vi "Answer.vi"(4 "连接ID":refnum<k5>, 6 "VISA串口名称":refnum<visa-resource-name>, 8 "error in (no error)":errorcluster caption="错误输入（无错误）", 9 "识别键":string, 10 "接收报文":string, 11 "MainPage 输入":refnum<class "MainPage.lvclass">) -> (0 "error out":errorcluster caption="错误输出", 3 "MainPage 输出":refnum<class "MainPage.lvclass">)   [LabVIEW 2019, in "MainPage.lvlib" / "MainPage.lvclass"]
uses:
  MainPage.lvclass
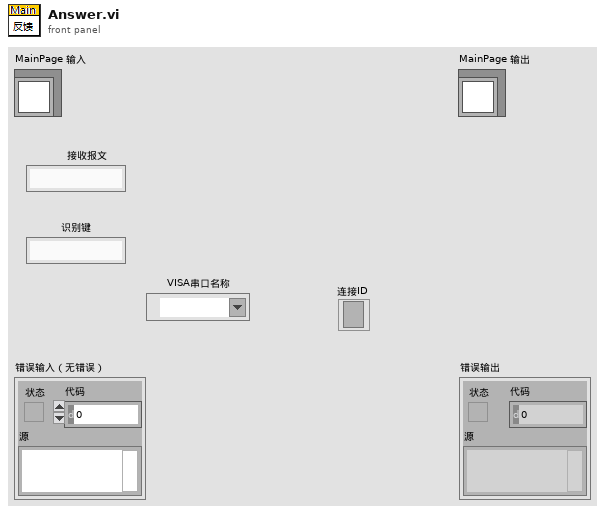
[diagram p1: front panel]
types:
  T1 = cluster{"类别":string, "通讯地址 U8":u8, "功能码 U8":u8, "寄存器地址 U16":u16, "数据/值 U16":u16, "16数据 U16":u16[]}
  T2 = cluster{"串口正常？":bool, "寄存器模拟":u16[], "报文信息记录":string[][]}
  T3 = enum16{"ini", "读取", "写入-报文记录", "写入-寄存器模拟", "写入-串口状态", "增加报文记录"}
  T4 = cluster{"寄存器模拟":u16[], "串口正常？":bool, "报文信息记录":string[][]}
  T5 = enum16{"ini", "增加记录", "读取记录", "更改寄存器值", "更改接口状态", "更改报文信息", "增加报文信息"}
  T6 = typedef "MainPage.lvlib/MainPage.lvclass/DataRef_通讯接口.ctl" = cluster{"连接方式":enum16{"网口(客服端)", "网口(服务端)", "串口"}, "VISA串口名称":refnum<visa-resource-name>, "服务端识别":cluster{"本机IP":string, "本机端口":u16, "当前目标":string}, "客服端识别":cluster{"客P-主IP:Port":string}, "服务端记录":cluster{"服务端侦听ID":refnum<k5>, "服务端接口记录":map{string, refnum<k5>}}, "客服端记录":map{string, refnum<k5>}}
  T7 = typedef "MainPage.lvlib/MainPage.lvclass/通用配置选项.ctl" = cluster{"ModBusRTU反馈":enum32{"模拟反馈", "无反馈", "错误反馈"}, "侦听周期":u32, "跳转反馈":bool, "报文记录数量":u16, "客服端新增模式":enum32{"单端模式", "多端共存"}}
  T8 = cluster{"类别":string, "通讯地址 U8":u8, "功能码 U8":u8, "03字节数 U8":u8, "03数据 U8":u8[], "6/16寄存器地址 U16":u16, "6/16数量/值 U16":u16}
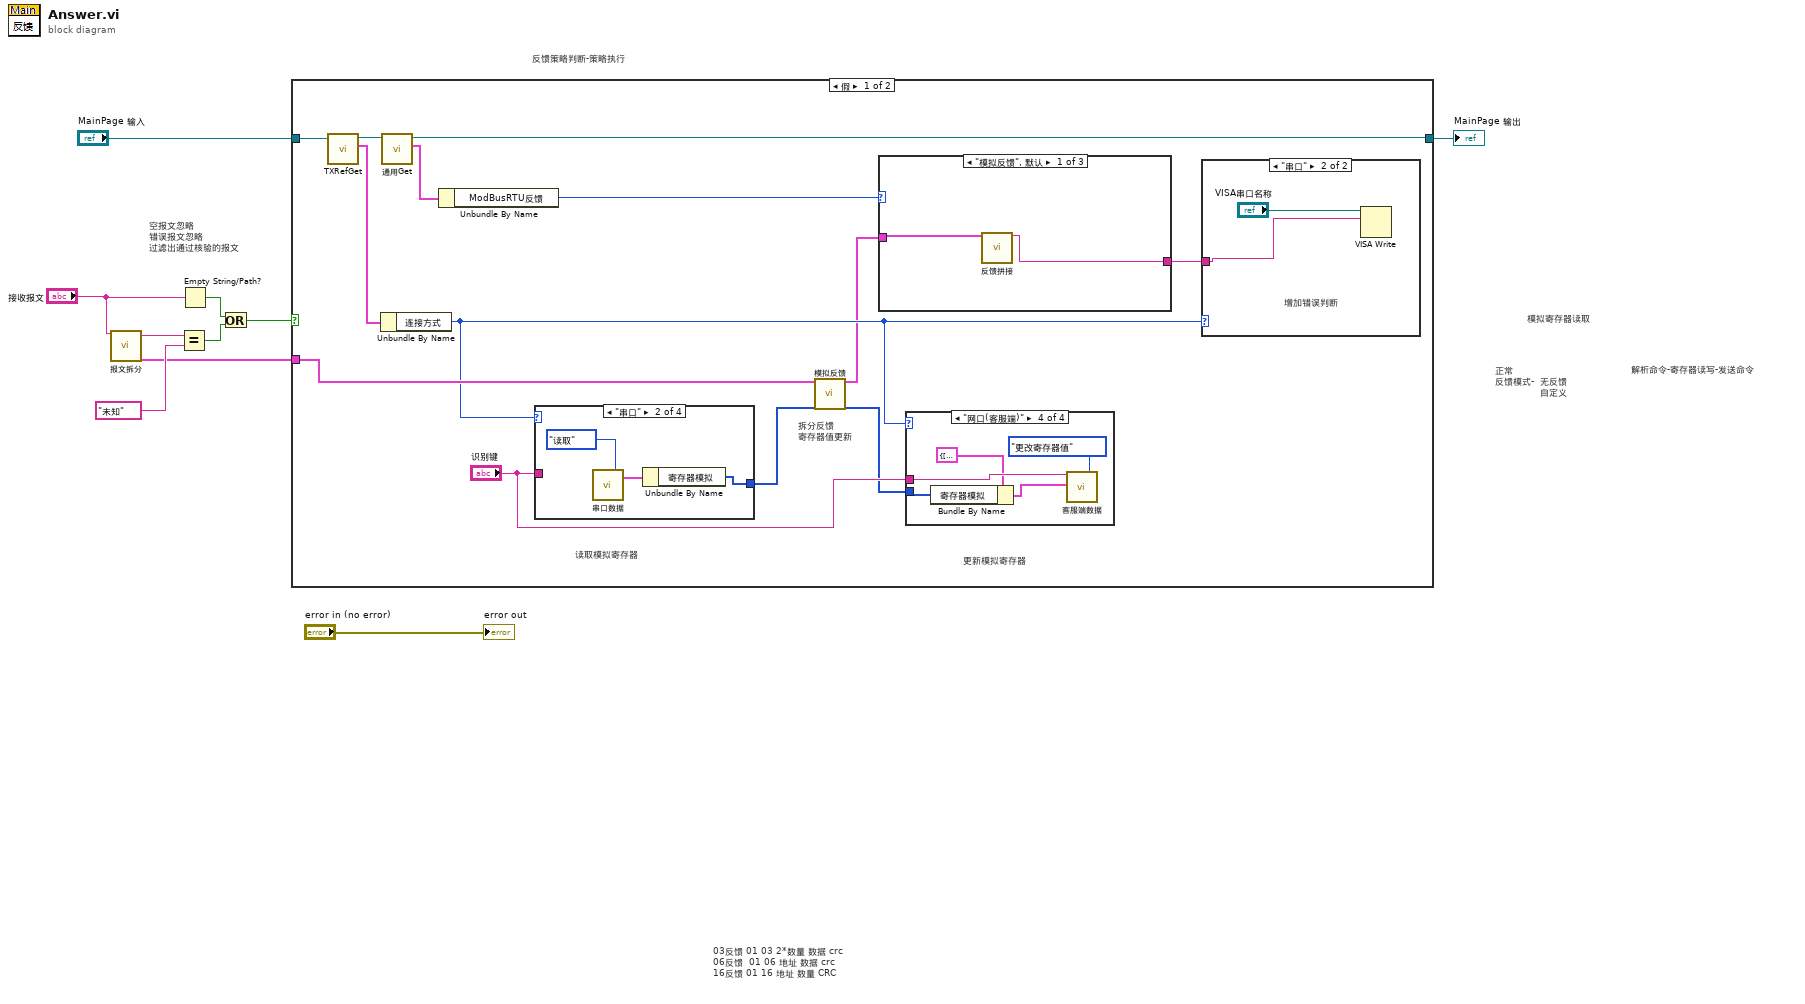
[diagram p0: block diagram]
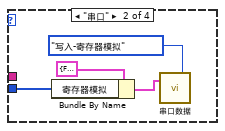
[diagram p3: hidden frame]
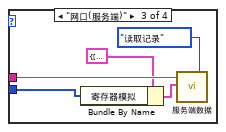
[diagram p4: hidden frame]
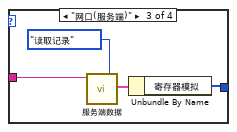
[diagram p6: hidden frame]
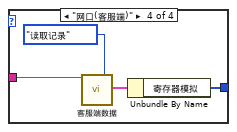
[diagram p7: hidden frame]
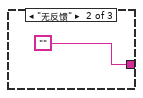
[diagram p8: hidden frame]
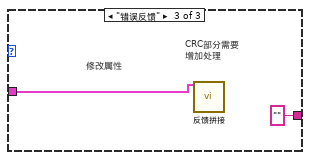
[diagram p9: hidden frame]
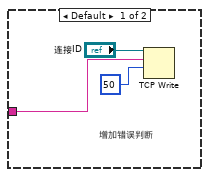
[diagram p10: hidden frame]
diagram:
  # "03反馈 01 03 2*数量 数据 crc\n06反馈  01 06 地址 数据 crc\n16反馈 01 16 地址 数量 CRC"
  # "解析命令-寄存器读写-发送命令"
  # "正常\n反馈模式-  无反馈\n               自定义"
  # "模拟寄存器读取"
  # "空报文忽略\n错误报文忽略\n过滤出通过核验的报文"
  # "反馈策略判断-策略执行"
  n1 = call "报文拆分.vi"("报文"="接收报文") -> ("类别"=w6:string, "拆分信息-数据"=w1:T1)  [unwired: 16 in, 1 out]
  n2 = Equal?(x=w6, y="未知" ("类别")) -> (x = y?=w3:bool)
  n3 = Empty String/Path?(string/path="接收报文") -> (empty?=w4:bool)
  n4 = Or(x=w4, y=w3) -> (x .or. y?=w2:bool)
  n5 = case shown="假" w2 {
    tunnel: [w20 w59] -> w9
    tunnel: "MainPage 输入" -> [w22 w59]
    tunnel: w1 -> [w17 _]
    frame False {
      # "更新模拟寄存器"
      # "拆分反馈\n寄存器值更新"
      # "读取模拟寄存器"
      n6 = call-dynamic "TXRefGet.vi"("MainPage 输入"=w22) -> ("通讯接口数据"=w23:T6, "MainPage 输出"=w21:refnum<class "MainPage.lvclass">)  [unwired: 6 in, 3 out]
      n7 = Unbundle By Name(w23) -> ("连接方式"=w13:enum16{"网口(客服端)", "网口(服务端)", "串口"})
      n8 = call-dynamic "通用Get.vi"("MainPage 输入"=w21) -> ("通用配置"=w19:T7, "MainPage 输出"=w20:refnum<class "MainPage.lvclass">)  [unwired: 6 in, 3 out]
      n9 = Unbundle By Name(w19) -> ("ModBusRTU反馈"=w18:enum32{"模拟反馈", "无反馈", "错误反馈"})
      n10 = case shown="\"串口\"" w13 {
        tunnel: "识别键" -> [_ _ w43 w47]
        tunnel: [_ w38 w41 w45] -> w16
        frame Default {
        }
        frame "串口" {
          n11 = call "串口数据.vi"("枚举"=T3."读取") -> ("串口记录"=w39:T2)  [unwired: 18 in]
          n12 = Unbundle By Name(w39) -> ("寄存器模拟"=w38:u16[])
        }
        frame "网口(服务端)" {
          n13 = call "服务端数据.vi"("IP-Port"=w43, "枚举"=T5."读取记录") -> ("数据获取"=w42:T4)  [unwired: 16 in, 1 out]
          n14 = Unbundle By Name(w42) -> ("寄存器模拟"=w41:u16[])
        }
        frame "网口(客服端)" {
          n15 = call "客服端数据.vi"("客P-主IP:P"=w47, "枚举"=T5."读取记录") -> ("数据获取"=w46:T4)  [unwired: 16 in, 1 out]
          n16 = Unbundle By Name(w46) -> ("寄存器模拟"=w45:u16[])
        }
      }
      n17 = call "模拟反馈.vi"("拆分信息-数据"=w17, "寄存器输入"=w16) -> ("反馈参数"=w12:T8, "寄存器输出"=w14:u16[])  [unwired: 16 in]
      n18 = case shown="\"模拟反馈\", 默认" w18 {
        tunnel: w12 -> [w50 _ w52]
        tunnel: [w49 "" ""] -> w11
        frame "模拟反馈", Default {
          n19 = call "反馈拼接.vi"("反馈参数"=w50) -> ("计算后字符串"=w49:string)  [unwired: 18 in]
        }
        frame "无反馈" {
        }
        frame "错误反馈" {
          # "CRC部分需要\n增加处理"
          # "修改属性"
          n20 = call "反馈拼接.vi"("反馈参数"=w52) -> ()  [unwired: 18 in, 1 out]
        }
      }
      n21 = case shown="\"网口(客服端)\"" w13 {
        tunnel: "识别键" -> [_ _ w31 w36]
        tunnel: w14 -> [_ w24 w28 w33]
        frame Default {
        }
        frame "串口" {
          n22 = Bundle By Name(cluster=T2 {"串口正常？"=FALSE, "寄存器模拟"=[], "报文信息记录"=[]} ("串口输入"), "寄存器模拟"=w24) -> (w25:T2)
          n23 = call "串口数据.vi"("串口输入"=w25, "枚举"=T3."写入-寄存器模拟") -> ()  [unwired: 17 in, 1 out]
        }
        frame "网口(服务端)" {
          n24 = Bundle By Name(cluster=T4 {"寄存器模拟"=[], "串口正常？"=FALSE, "报文信息记录"=[]} ("数据输入"), "寄存器模拟"=w28) -> (w29:T4)
          n25 = call "服务端数据.vi"("IP-Port"=w31, "数据输入"=w29, "枚举"=T5."读取记录") -> ()  [unwired: 15 in, 2 out]
        }
        frame "网口(客服端)" {
          n26 = Bundle By Name(cluster=T4 {"寄存器模拟"=[], "串口正常？"=FALSE, "报文信息记录"=[]} ("数据输入"), "寄存器模拟"=w33) -> (w34:T4)
          n27 = call "客服端数据.vi"("客P-主IP:P"=w36, "数据输入"=w34, "枚举"=T5."更改寄存器值") -> ()  [unwired: 15 in, 2 out]
        }
      }
      n28 = case shown="\"串口\"" w13 {
        tunnel: w11 -> [w55 w57]
        frame Default {
          # "增加错误判断"
          n29 = TCP Write(connection ID="连接ID", data in=w55, 9:50 ("超时毫秒(25000)")) -> ()  [unwired: 1 in, 3 out]
        }
        frame "串口" {
          # "增加错误判断"
          n30 = VISA Write(VISA resource name="VISA串口名称", write buffer=w57) -> ()  [unwired: 1 in, 3 out]
        }
      }
    }
    frame True {
    }
  }
  "MainPage 输出" <- w9
  "error out" <- "error in (no error)"
